vi "PIDF.vi"(0 "setpoint":dbl format="%.2f", 1 "output range":cluster{"output high":dbl, "output low":dbl}={"output high"=1.0, "output low"=-1.0} {"output low" format="%.2f"; "output high" format="%.2f"}, 3 "invert? (F)":bool, 5 "process variable":dbl format="%.2f", 7 "Allowed Error":dbl, 9 "Feedforward":dbl, 11 "i Zone":dbl=inf format="%.2f", 12 "PIDF gains":cluster{"Kp":dbl, "Ki":dbl, "Kd":dbl, "Kf":dbl} {"Kf" format="%.3f"; "Kd" format="%.3f"; "Ki" format="%.3f"; "Kp" format="%.3f"}, 14 "reinitialize? (F)":bool) -> (4 "output":dbl format="%.2f", 6 "In Range?":bool, 10 "In i Zone?":bool)   [LabVIEW 2018]
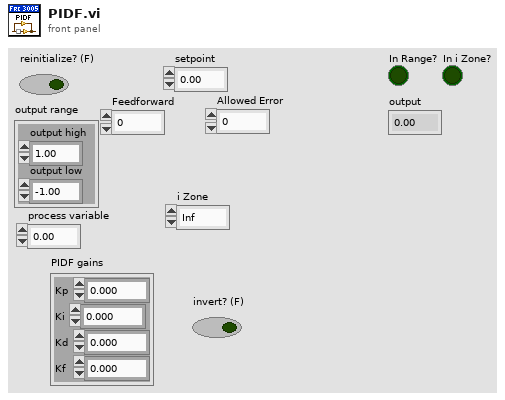
[diagram p1: front panel]
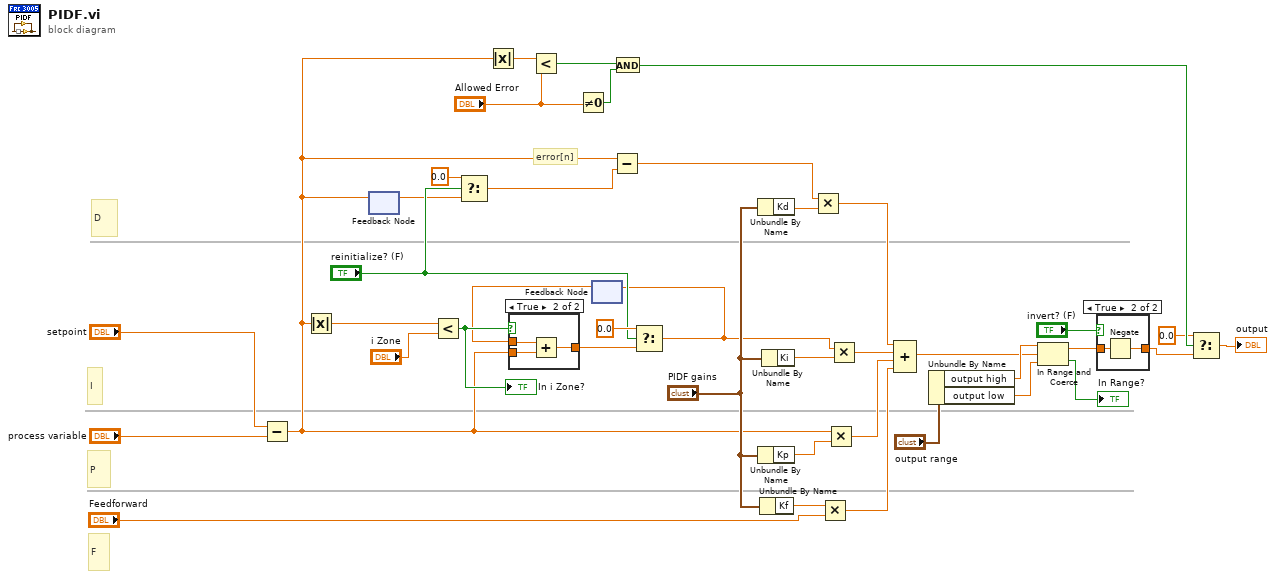
[diagram p0: block diagram]
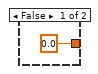
[diagram p3: hidden frame]
diagram:
  # "F"
  # "D"
  # "I"
  # "P"
  # "error[n]"
  n1 = Subtract(x="setpoint", y="process variable") -> (x-y=w9:dbl)
  n2 = Absolute Value(x=w9) -> (abs(x)=w38:dbl)
  n3 = feedback #1() -> (w30:dbl)  [unwired: 1 in]
  n4 = feedback-in #1(w9) -> ()
  n5 = Less?(x=w38, y="i Zone") -> (x < y?=w36:bool)
  "In i Zone?" <- w36
  n6 = Select(t=0.0 ("f"), s="reinitialize? (F)", f=w30) -> (s? t:f=w29:dbl)
  n7 = Absolute Value(x=w9) -> (abs(x)=w8:dbl)
  n8 = Less?(x=w8, y="Allowed Error") -> (x < y?=w5:bool)
  n9 = Not Equal To 0?(x="Allowed Error") -> (x != 0?=w6:bool)
  n10 = feedback #2() -> (w35:dbl)  [unwired: 1 in]
  n11 = case shown="True" w36 {
    tunnel: w9 -> [_ w44]
    tunnel: [0.0 ("f") w43] -> w34
    tunnel: w35 -> [_ w42]
    frame False {
    }
    frame True {
      n12 = Add(x=w42, y=w44) -> (x+y=w43:dbl)
    }
  }
  n13 = Subtract(x=w9, y=w29) -> (x-y=w19:dbl)
  n14 = And(x=w5, y=w6) -> (x .and. y?=w4:bool)
  n15 = Select(t=0.0 ("f"), s="reinitialize? (F)", f=w34) -> (s? t:f=w16:dbl)
  n16 = feedback-in #2(w16) -> ()
  n17 = Unbundle By Name("PIDF gains") -> ("Kd"=w20:dbl)
  n18 = Unbundle By Name("PIDF gains") -> ("Kp"=w39:dbl)
  n19 = Unbundle By Name("PIDF gains") -> ("Kf"=w22:dbl)
  n20 = Unbundle By Name("PIDF gains") -> ("Ki"=w17:dbl)
  n21 = Multiply(x=w19, y=w20) -> (x*y=w18:dbl)
  n22 = Multiply(x=w22, y="Feedforward") -> (x*y=w21:dbl)
  n23 = Multiply(x=w9, y=w39) -> (x*y=w28:dbl)
  n24 = Multiply(x=w16, y=w17) -> (x*y=w15:dbl)
  n25 = Compound Arithmetic op=ADD(w18, w15, w28, w21) -> (w24:dbl)
  n26 = Unbundle By Name("output range") -> ("output high"=w26:dbl, "output low"=w25:dbl)
  n27 = In Range and Coerce(upper limit=w26, x=w24, lower limit=w25) -> (coerced(x)=w13:dbl, In Range?=→"In Range?":bool)
  n28 = case shown="True" "invert? (F)" {
    tunnel: w13 -> [w45 w47]
    tunnel: [w45 w46] -> w2
    frame False {
    }
    frame True {
      n29 = Negate(x=w47) -> (-x=w46:dbl)
    }
  }
  n30 = Select(t=0.0, s=w4, f=w2) -> (s? t:f=→"output":dbl)
